vi "Square Waveform.vi"(4 "duty cycle (%)":dbl=50.0 format="%0.2f", 5 "offset":dbl format="%0.2p", 6 "sampling info":cluster{"Fs":dbl, "#s":dbl}={"Fs"=1000.0, "#s"=1000.0} {"Fs" format="%.2p"}, 7 "reset signal":bool, 8 "error in (no error)":errorcluster, 9 "phase":dbl format="%.2p", 10 "amplitude":dbl=1.0 format="%0.2p", 11 "frequency":dbl=10.0 format="%0.2p") -> (0 "error out":errorcluster, 3 "signal out":waveform(dbl))   [LabVIEW 2009]
doc: "Generates a waveform containing a square wave."
uses:
  ma_Updatet0 timestamp.vi
  <vilib>/measure/NI_MABase.lvlib
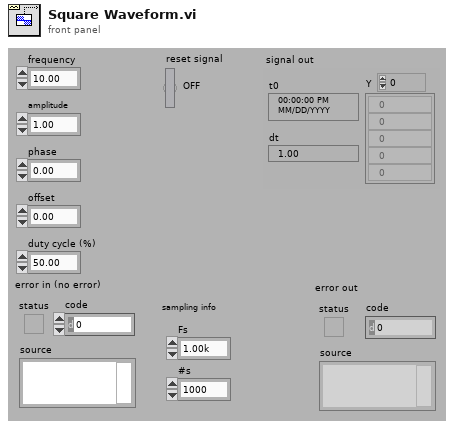
[diagram p1: front panel]
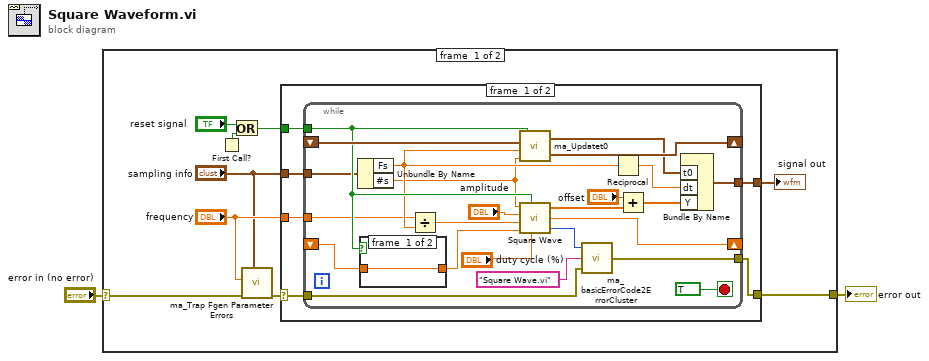
[diagram p0: block diagram]
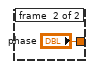
[diagram p2: hidden frame]
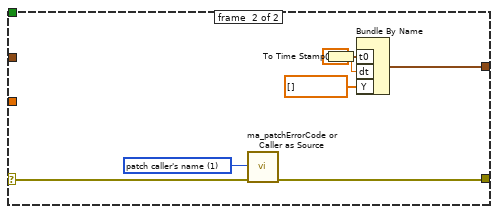
[diagram p3: hidden frame]
diagram:
  n1 = case shown="No Error" "error in (no error)" {
    selector: "error in (no error)" -> [w3 w51]
    tunnel: [w7 w51] -> w2
    frame #0 {
      n2 = First Call?() -> (First Call?: T/F=w4:bool)
      n3 = Or(x="reset signal", y=w4) -> (x .or. y?=w10:bool)
      n4 = call "ma_Trap Fgen Parameter Errors.vi"("Sampling info"="sampling info", "error in (no error)"=w3, "frequency"="frequency") -> ("error out"=w9:errorcluster)  [unwired: 8 in]
      n5 = case shown="No Error" w9 {
        selector: w9 -> [w12 w46]
        tunnel: w10 -> [w17 _]
        tunnel: "sampling info" -> [w16 _]
        tunnel: "frequency" -> [w15 _]
        tunnel: [w14 w45] -> w7
        tunnel: [w13 w48] -> w5
        frame #0 {
          n6 = while {
            tunnel: w12 -> [w19]
            tunnel: [w21] -> w13
            tunnel: [w22] -> w14
            tunnel: w15 -> [w23]
            tunnel: w16 -> [w24]
            tunnel: w17 -> [w28]
            shift-left: _ -> [w31]
            shift-right: [w33] -> _
            shift-left: _ -> [w38]
            shift-right: [w37] -> _
            stop <- TRUE stop-if-true
            n7 = Unbundle By Name(w24) -> ("Fs"=w26:dbl, "#s"=w25:dbl)
            n8 = case shown="True" w28 {
              tunnel: [w42 "phase"] -> w32
              tunnel: w31 -> [w42 _]
              frame #0 {
              }
              frame #1 {
              }
            }
            n9 = Divide(x=w23, y=w26) -> (x/y=w27:dbl)
            n10 = call-poly "ma_Updatet0.vi"("samples"=w25, "sampling rate (S/s)"=w26, "tf previous"=w38, "Reset Generation"=w28) -> ("tf new"=w37:timestamp, "t0"=w18:timestamp)
            n11 = call "Square Wave.vi"("samples"=w25, "reset phase"=w28, "amplitude"="amplitude", "f"=w27, "duty cycle (%)"="duty cycle (%)", "phase in"=w32) -> ("square wave"=w35:dbl[], "phase out"=w33:dbl, "error"=w41:i32)
            n12 = call <vilib>:"ma_basicErrorCode2ErrorCluster.vi"("error in (no error)"=w19, "subVI name"="Square Wave.vi" ("subVI Name"), "Error Code"=w41) -> ("error out"=w22:errorcluster)
            n13 = Reciprocal(x=w26) -> (1/x=w30:dbl)
            n14 = Add(x="offset", y=w35) -> (x+y=w34:dbl[])
            n15 = Bundle By Name("t0"=w18, "dt"=w30, "Y"=w34) -> (w21:waveform(dbl))  [unwired: 1 in]
          }
        }
        frame #1 {
          w44 = u16 1 items=["patch error code", "patch caller's name"] ("operation")
          w50 = 0.0 ("t0")
          n16 = call "ma_patchErrorCode or Caller as Source.vi"("error in (no error)"=w46, "operation"=w44) -> ("error out"=w45:errorcluster)  [unwired: 9 in]
          n17 = To Time Stamp(1:w50) -> (0:w47:timestamp)
          n18 = Bundle By Name("t0"=w47, "dt"=w50, "Y"=dbl[] []) -> (w48:waveform(dbl))  [unwired: 1 in]
        }
      }
      "signal out" <- w5
    }
    frame #1 {
    }
  }
  "error out" <- w2
